vi "DO Post Step Type.vi"(8 "error in (no error)":errorcluster, 9 "DOWrite":T1, 10 "Socket No":u16=1, 11 "DO in":refnum<class "DO.lvclass">) -> (0 "error out":errorcluster, 2 "PhysicalChannel":string[](array[string]), 3 "DO out":refnum<class "DO.lvclass">)   [LabVIEW 2023, in "HardwareAbstractionLayer_LVOOP.lvlib" / "DO.lvclass"]
uses:
  DO.lvclass
  Control/DO Write Enable.ctl
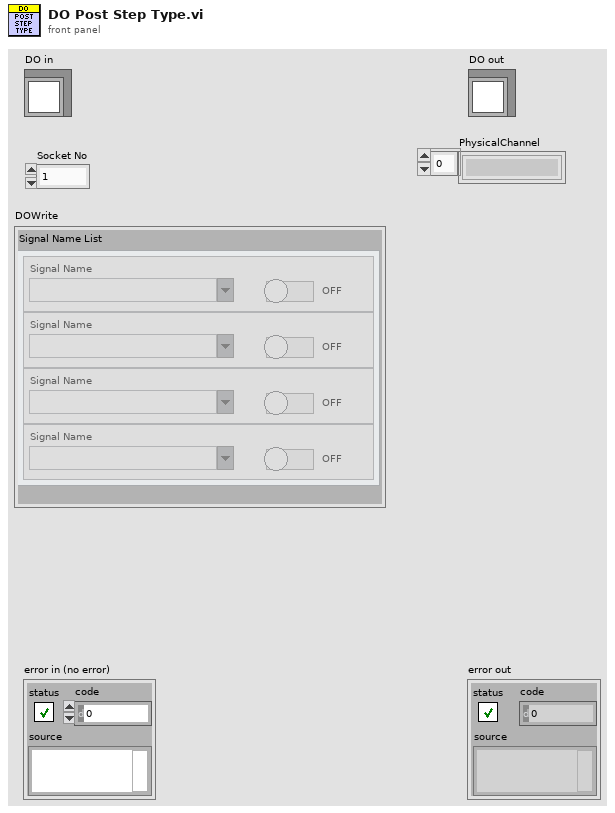
[diagram p1: front panel]
types:
  T1 = typedef "HardwareAbstractionLayer_LVOOP.lvlib/DO.lvclass/DO Write Enable.ctl" = cluster{"Signal Name List":cluster{"Signal Name":string, "Enable Output":bool}[]}
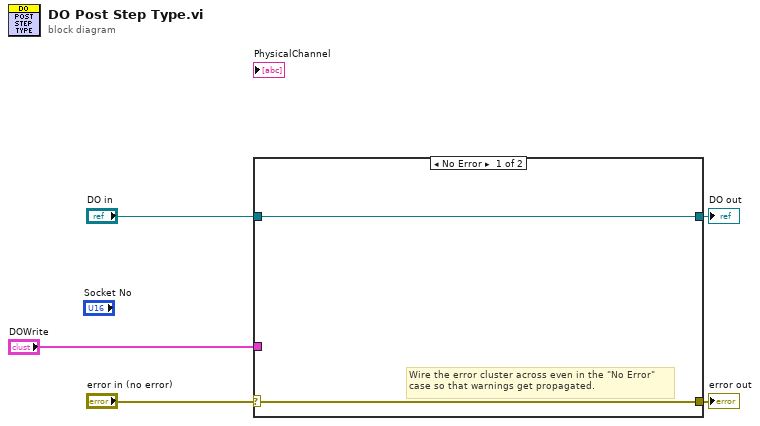
[diagram p0: block diagram]
diagram:
  n1 = case shown="No Error" "error in (no error)" {
    selector: "error in (no error)" -> [w7 w9]
    tunnel: [w7 w9] -> w4
    tunnel: [w6 w8] -> w2
    tunnel: "DO in" -> [w6 w8]
    tunnel: "DOWrite" -> [_ _]
    frame No Error {
      # "Wire the error cluster across even in the \"No Error\"\ncase so that warnings get propagated."
    }
    frame Error {
    }
  }
  "error out" <- w4
  "DO out" <- w2
